vi "Motor Loop.vi"(8 "error in":errorcluster) -> (0 "error out":errorcluster)   [LabVIEW 2011]
uses:
  Utilities/Robot Parameters/Robot Parameters.vi
  <vilib>/Platform/TimedLoop/XDataNode/XDataNode.xnode
  <vilib>/Platform/TimedLoop/XDataNode/nitl_modes.ctl
  <vilib>/Platform/TimedLoop/XDataNode/XDNodeRunTimeDep.lvlib
  <vilib>/Platform/TimedLoop/XDataNode/wakeup.ctl
  <vilib>/Platform/TimedLoop/XDataNode/timing_clust.ctl
  <vilib>/robotics/Steering/Steering Frame/Apply Velocity to Motors.vi
  <vilib>/robotics/Steering/Steering Frame/NI_Robotics_Steering Frame.lvclass
  <vilib>/Simulation/Implementation/XNodeFramework/SimXNode/SimX.xnode
  <vilib>/robotics/Steering/Steering Frame/Get Velocity from Motors.vi
  <vilib>/Simulation/Implementation/Shared/SIMSCR Execution Mode.ctl
  <vilib>/Simulation/Scripting/Companion Diagram/SimConfigNode/_simSolvers.ctl
  <vilib>/Simulation/Scripting/Companion Diagram/SimConfigNode/SimParams.ctl
  <vilib>/Simulation/Scripting/Companion Diagram/SimConfigNode/SimDog.xnode
  <vilib>/Simulation/Utility/Implementation/SIM Halt.vi
  <vilib>/Simulation/Model Libraries/PID/SIM PID.vi
  <vilib>/Simulation/Nonlinear/Implementation/NILVSim Saturation.llb/SIM Saturation (scalar).vi
  <vilib>/Simulation/Model Libraries/PID/SIM PID (Parallel).vi
  <vilib>/robotics/Steering/Steering Frame/Get Steering Frame Velocity from Motors.vi
  <vilib>/robotics/Steering/Steering Frame/Apply Steering Frame Velocity to Motors.vi
  <vilib>/Simulation/Nonlinear/Implementation/NILVSim Saturation.llb/SIM Saturation (vector).vi
  <vilib>/robotics/Utilities/NI_Robotics Utilities.lvlib
  <vilib>/Analysis/coordinate.llb/2D Cartesian Coordinate Rotation.vi
  <vilib>/Analysis/NI_AALPro.lvlib
  <vilib>/Analysis/coordinate.llb/2D Cartesian Coordinate Rotation (Scalar).vi
  <vilib>/Simulation/ContinuousLinear/Implementation/NILVSim Integrator new.llb/SIM Integrator (vector).vi
  <vilib>/Simulation/ContinuousLinear/Implementation/NILVSim Integrator new.llb/SIM Integrator (scalar).vi
panel:
  out "Telemetry":T1={"Voltage"={0.0, 0.0, 0.0}, "Encoder Speed"={0, 0}, "Temps"={"IC Temp (C)"=0, "Ch1 Temp (C)"=0, "Ch2 Temp (C)"=0}, "Current"={0.0, 0.0, 0.0, 4.6238981750249924e+36}} {"Current" scale=0.0..16.0; "Temps"."IC Temp (C)" scale=0.0..150.0; "Temps"."Ch1 Temp (C)" scale=0.0..150.0; "Temps"."Ch2 Temp (C)" scale=0.0..150.0; "Encoder Speed" scale=-100.0..100.0; "Voltage" scale=8.0..14.0}
  in  "VISA resource name":refnum<visa-resource-name>
  in  "Debug":bool
  out "Command to Serial":string
  in  "End Loop":bool
  in  "stop?":bool
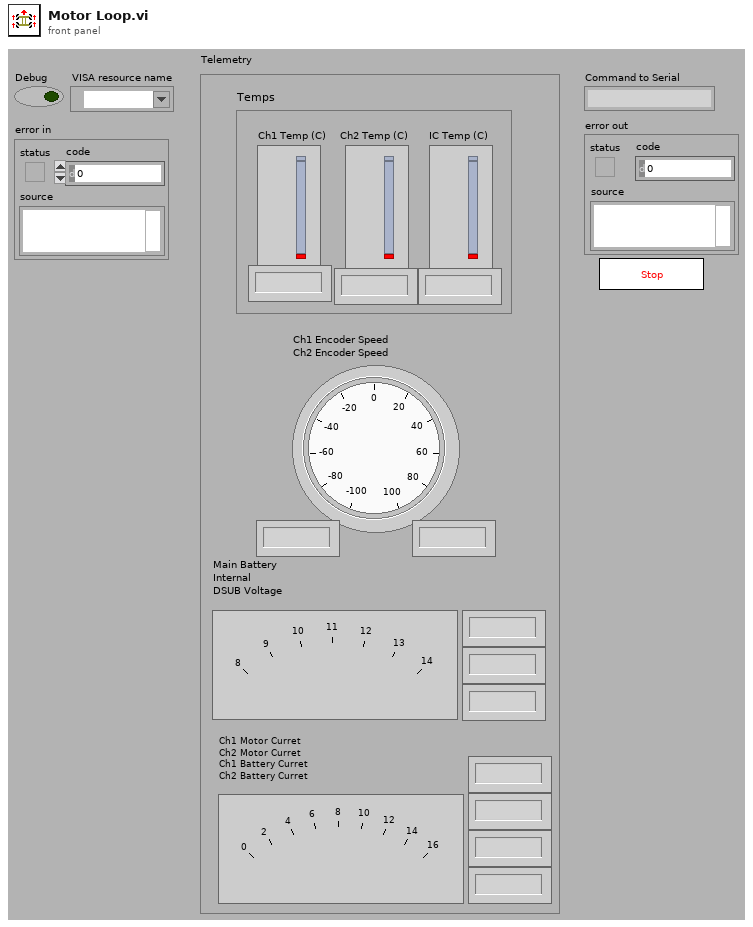
[diagram p1: front panel]
types:
  T1 = cluster{"Voltage":cluster{sgl, sgl, sgl}, "Encoder Speed":cluster{i32, i32}, "Temps":cluster{"IC Temp (C)":i32, "Ch1 Temp (C)":i32, "Ch2 Temp (C)":i32}, "Current":cluster{dbl, dbl, dbl, dbl}}
  T2 = typedef "XDNodeRunTimeDep.lvlib/timing_clust.ctl" = cluster{"Expected End [f-1]":u64, "Actual End [f-1]":u64, "Finished Late? [f-1]":bool, "Expected End [i-1]":u64, "Actual End [i-1]":u64, "Finished Late? [i-1]":bool, "Expected Start [i]":u64, "Actual Start [i]":u64, "Expected Start [f]":u64, "Actual Start [f]":u64, "Source Name":string, "Structure Name":string, "Period":i64, "Deadline":i64, "Offset":i64, "Start":i64, "Priority":i32, "Timeout":i32, "Mode":T3, "Wakeup Reason":T4, "Error":errorcluster, "Source Type":string, "Secondary Source Type":string, "Global End Time":u64, "Global Start Time":u64, "Frame Duration":u64, "Iteration Duration":u64, "Assigned CPU":i32, "I/O Scan Engine Mode":u32}
  T3 = typedef "XDNodeRunTimeDep.lvlib/nitl_modes.ctl" = enum32{"No Change", "Process missed periods, maintain original phase", "Discard missed periods, maintain original phase", "Process missed periods, ignore original phase", "Discard missed periods, ignore original phase"}
  T4 = typedef "XDNodeRunTimeDep.lvlib/wakeup.ctl" = enum32{"Normal", "Aborted", "Asynchronous wakeup", "Timing source error", "Timed loop error", "Timeout"}
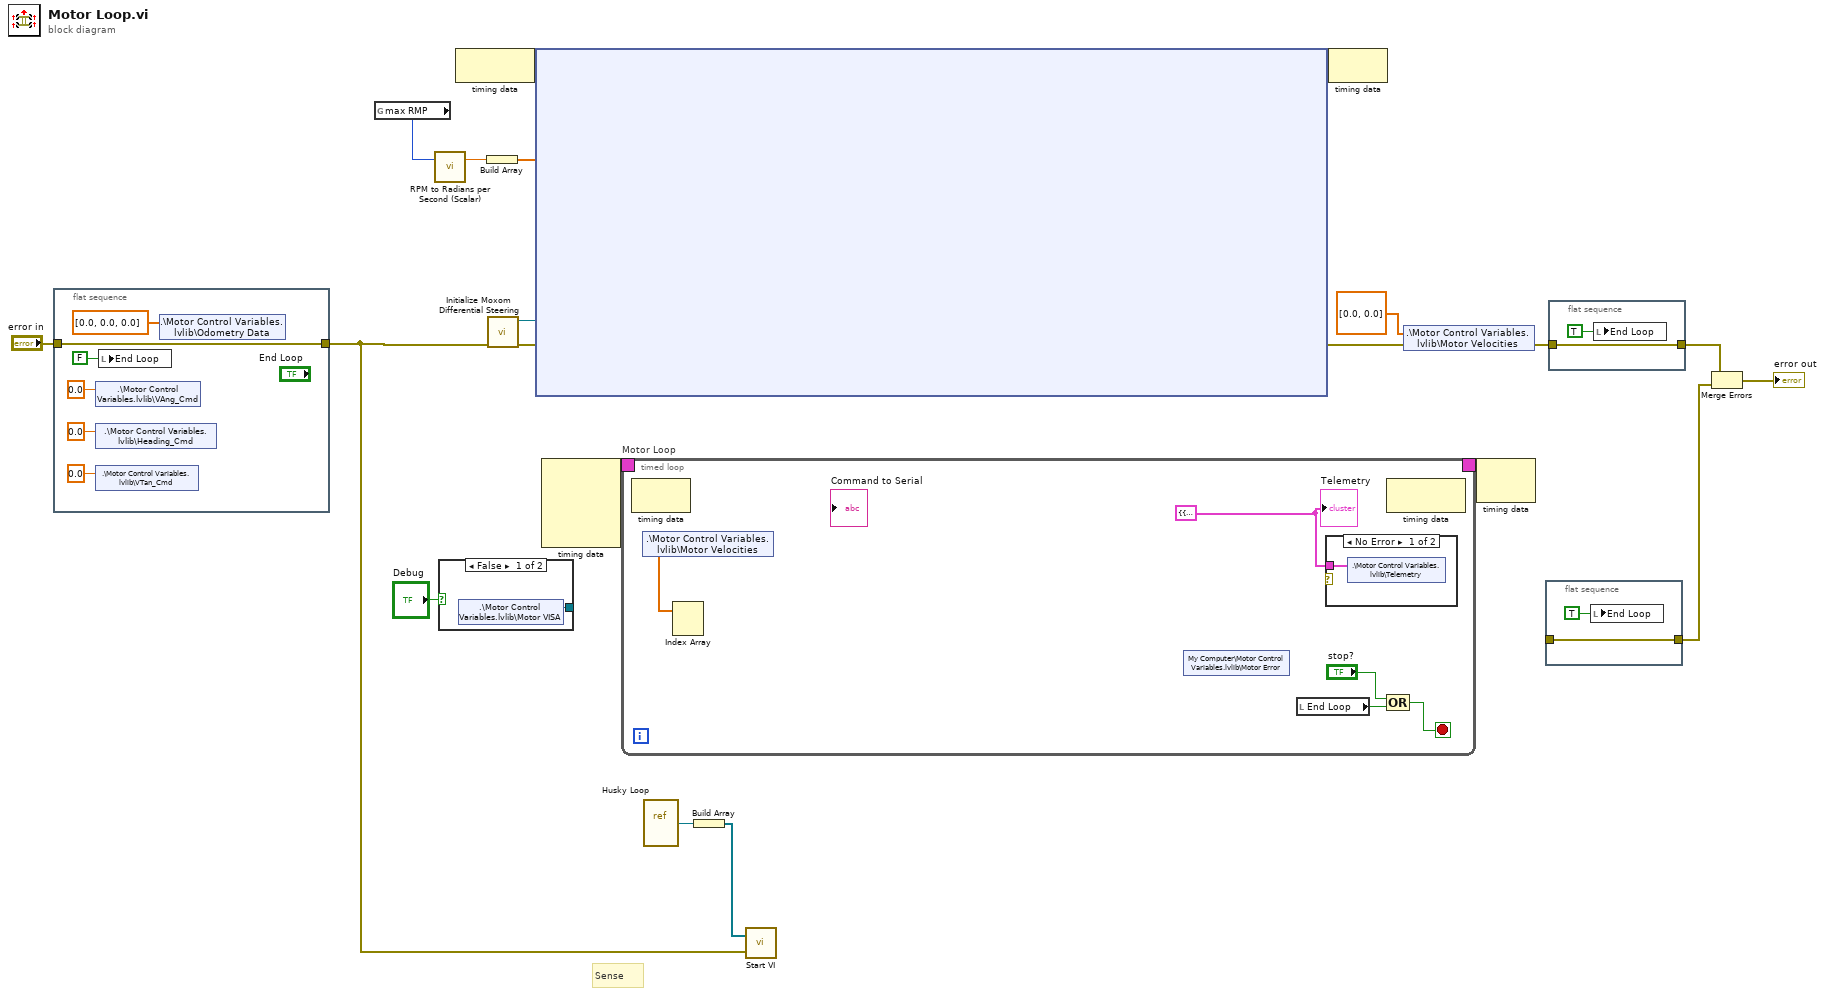
[diagram p0: block diagram]
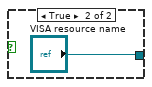
[diagram p2: hidden frame]
diagram:
  # "Sense"
  n1 = flat-sequence {
    tunnel: [w22] -> w1
    tunnel: "error in" -> [w22]
    frame #0 {
      n2 = shared-variable ".\\Motor Control Variables.lvlib\\VAng_Cmd"(0.0 ("VX_Cmd")) -> ()  [unwired: 1 in, 1 out]
      n3 = shared-variable ".\\Motor Control Variables.lvlib\\Heading_Cmd"(0.0 ("Heading_Cmd")) -> ()  [unwired: 1 in, 1 out]
      n4 = shared-variable ".\\Motor Control Variables.lvlib\\VTan_Cmd"(0.0 ("VY_Cmd")) -> ()  [unwired: 1 in, 1 out]
      n5 = local write "End Loop"(FALSE ("End Loop")) -> ()
      n6 = shared-variable ".\\Motor Control Variables.lvlib\\Odometry Data"(dbl[] [0.0, 0.0, 0.0] ("Odometry Data")) -> ()  [unwired: 1 in, 1 out]
    }
  }
  n7 = global read "Robot Parameters.vi" "max RMP"() -> (w4:i32)
  n8 = call <vilib>:"RPM to Radians per Second (Scalar).vi"("rpm"=w4) -> ("radians per second"=w10:dbl)  [unwired: 2 in]
  n9 = case shown="False" "Debug" {
    tunnel: [w27 "VISA resource name"] -> _
    frame False {
      n10 = shared-variable ".\\Motor Control Variables.lvlib\\Motor VISA"() -> (w27:refnum<visa-resource-name>)  [unwired: 1 in, 1 out]
    }
    frame True {
    }
  }
  n11 = node-c288() -> (w16:variant)  [unwired: 1 in]
  n12 = Build Array(w10) -> (w9:dbl[])
  n13 = call "Initialize Moxom Differential Steering.vi"("error in (no error)"=w1) -> ("error out"=w7:errorcluster, "differential steering frame out"=w8:refnum<class "NI_Robotics_Differential Steering Frame.lvclass">)  [unwired: 9 in]
  n14 = node-c254 ("Simulation Loop 3")(w16, w9, w7, w8) -> (w15:variant, w6:errorcluster)
  n15 = node-c288() -> (w18:T2)  [unwired: 4 in]
  n16 = timed-loop "Motor Loop" {
    timing: w18 -> [_]
    timing-out: [_] -> w17
    stop <- w32 stop-if-true
    w29 = T1 {"Voltage"={0.0, 0.0, 0.0}, "Encoder Speed"={0, 0}, "Temps"={"IC Temp (C)"=0, "Ch1 Temp (C)"=0, "Ch2 Temp (C)"=0}, "Current"={0.0, 0.0, 0.0, 0.0}} ("Telemetry")
    n17 = node-c288() -> ()  [unwired: 1 in, 1 out]
    n18 = shared-variable ".\\Motor Control Variables.lvlib\\Motor Velocities"() -> (w30:dbl[])  [unwired: 1 in, 1 out]
    n19 = Index Array(array=w30) -> ()  [unwired: 2 in, 2 out]
    n20 = shared-variable "My Computer\\Motor Control Variables.lvlib\\Motor Error"() -> ()  [unwired: 2 in, 1 out]
    n21 = local read "End Loop"() -> (w31:bool)
    n22 = case shown="No Error" {
      selector: _ -> [_ _]
      tunnel: w29 -> [w36 _]
      frame No Error {
        n23 = shared-variable ".\\Motor Control Variables.lvlib\\Telemetry"(w36) -> ()  [unwired: 1 in, 1 out]
      }
      frame Error {
      }
    }
    n24 = node-c288() -> ()  [unwired: 1 in, 1 out]
    n25 = Compound Arithmetic op=OR("stop?", w31) -> (w32:bool)
    "Telemetry" <- w29
  }
  n26 = vi-ref "Husky Loop.vi"() -> (w2:refnum<vi>)
  n27 = Build Array(w2) -> (w3:refnum<vi>[])
  n28 = call "Start VI.vi"("error in"=w1, "VI refnum"=w3) -> ()  [unwired: 1 in, 1 out]
  n29 = node-c288(w15) -> ()  [unwired: 1 out]
  n30 = shared-variable ".\\Motor Control Variables.lvlib\\Motor Velocities"(dbl[] [0.0, 0.0] ("Motor Velocities"), error in=w6) -> (error out=w11:errorcluster)
  n31 = node-c288(w17) -> ()  [unwired: 1 out]
  n32 = flat-sequence {
    tunnel: _ -> [w37]
    tunnel: [w37] -> w13
    frame #0 {
      n33 = local write "End Loop"(TRUE ("End Loop")) -> ()
    }
  }
  n34 = flat-sequence {
    tunnel: [w39] -> w12
    tunnel: w11 -> [w39]
    frame #0 {
      n35 = local write "End Loop"(TRUE ("End Loop")) -> ()
    }
  }
  n36 = Merge Errors(w12, w13) -> (→"error out":errorcluster)
